vi "Image Validity FGV.vi"(7 "Image Validity FGV_Commands":T1, 8 "Error In":errorcluster, 11 "Validity status IN":bool) -> (0 "Error Out":errorcluster, 3 "Validity status OUT":bool)   [LabVIEW 2012]
doc: "SciScan 1.2 160622"
uses:
  Image Validity FGV_Commands.ctl
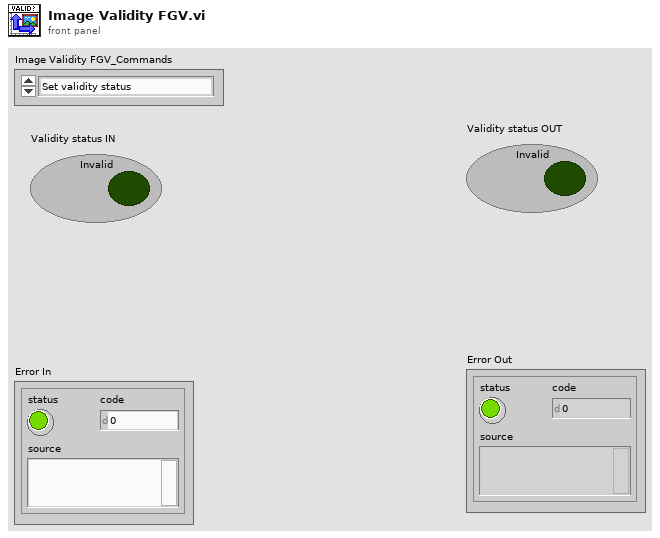
[diagram p1: front panel]
types:
  T1 = typedef "Image Validity FGV_Commands.ctl" = enum16{"Set validity status", "Get Validity status"}
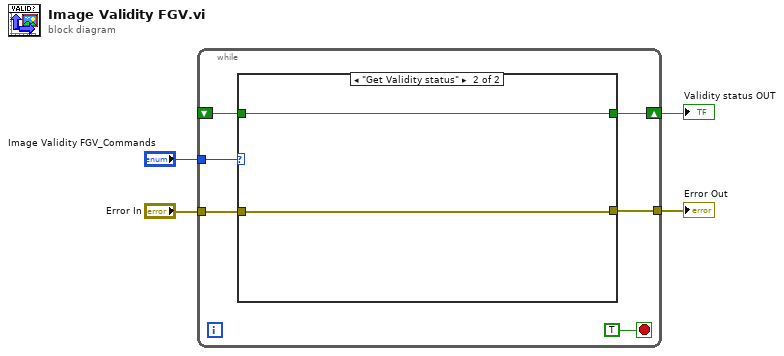
[diagram p0: block diagram]
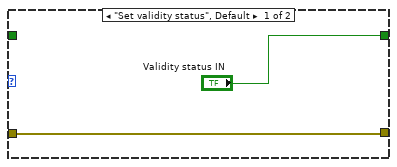
[diagram p2: hidden frame]
diagram:
  n1 = while {
    tunnel: "Image Validity FGV_Commands" -> [w9]
    shift-right: [w8] -> w3
    shift-left: _ -> [w7]
    tunnel: "Error In" -> [w6]
    tunnel: [w5] -> w1
    stop <- TRUE stop-if-true
    n2 = case shown="\"Get Validity status\"" w9 {
      tunnel: ["Validity status IN" w14] -> w8
      tunnel: w7 -> [_ w14]
      tunnel: [w11 w13] -> w5
      tunnel: w6 -> [w11 w13]
      frame "Set validity status", Default {
      }
      frame "Get Validity status" {
      }
    }
  }
  "Error Out" <- w1
  "Validity status OUT" <- w3
